vi "Create DSF UDP Loopback Configuration Files.vi"() -> ()   [LabVIEW 2021]
uses:
  Includes/DSF Core.lvlibp/Typedefs/DSF Timing Info.ctl
  Includes/DSF Core.lvlibp/Typedefs/DSF Settings Info.ctl
  Includes/DSF Core.lvlibp/Typedefs/DSF Engine Plugin Thread Configuration.ctl
  Includes/DSF Core.lvlibp/Typedefs/DSF Direction.ctl
  Includes/DSF Core.lvlibp/Typedefs/DSF Byte Order.ctl
  Includes/DSF Core.lvlibp/Typedefs/DSF Data Type.ctl
  Includes/DSF Core.lvlibp/Typedefs/DSF Engine Channel Configuration.ctl
  Includes/DSF Core.lvlibp/Typedefs/DSF Engine Transfer Configuration.ctl
  Includes/DSF Core.lvlibp/Typedefs/DSF Timeout Behavior.ctl
  Includes/DSF Core.lvlibp/Typedefs/DSF Engine Transfer Group Configuration.ctl
  Includes/DSF Core.lvlibp/Typedefs/DSF Engine Plugin Configuration.ctl
  Includes/DSF Core.lvlibp/Typedefs/DSF Engine Framework Configuration.ctl
  Includes/DSF Core.lvlibp/Typedefs/Core Channel Configuration.ctl
  Includes/DSF Core.lvlibp/Typedefs/Core Transfer Configuration.ctl
  Includes/DSF Core.lvlibp/Typedefs/Core Group Configuration.ctl
  Includes/DSF Core.lvlibp/Typedefs/Core Thread Configuration.ctl
  Includes/DSF Core.lvlibp/Typedefs/Core Plugin Configuration.ctl
panel:
  in  "Tx Ports":u16[](array[numeric])
  in  "Rx Ports":u16[](array[numeric])
  out "Framework Configuration":T1
  in  "channels data type":T16=enum."SGL"
  in  "channel count per transfer":u64=1000
  in  "Destination IP Address":string="localhost"
  in  "Source IP Address":string="localhost"
  in  "Local Ports":u16[](array[numeric])
  out "error out":errorcluster
  in  "error in (no error)":errorcluster
  in  "Output Folder":path
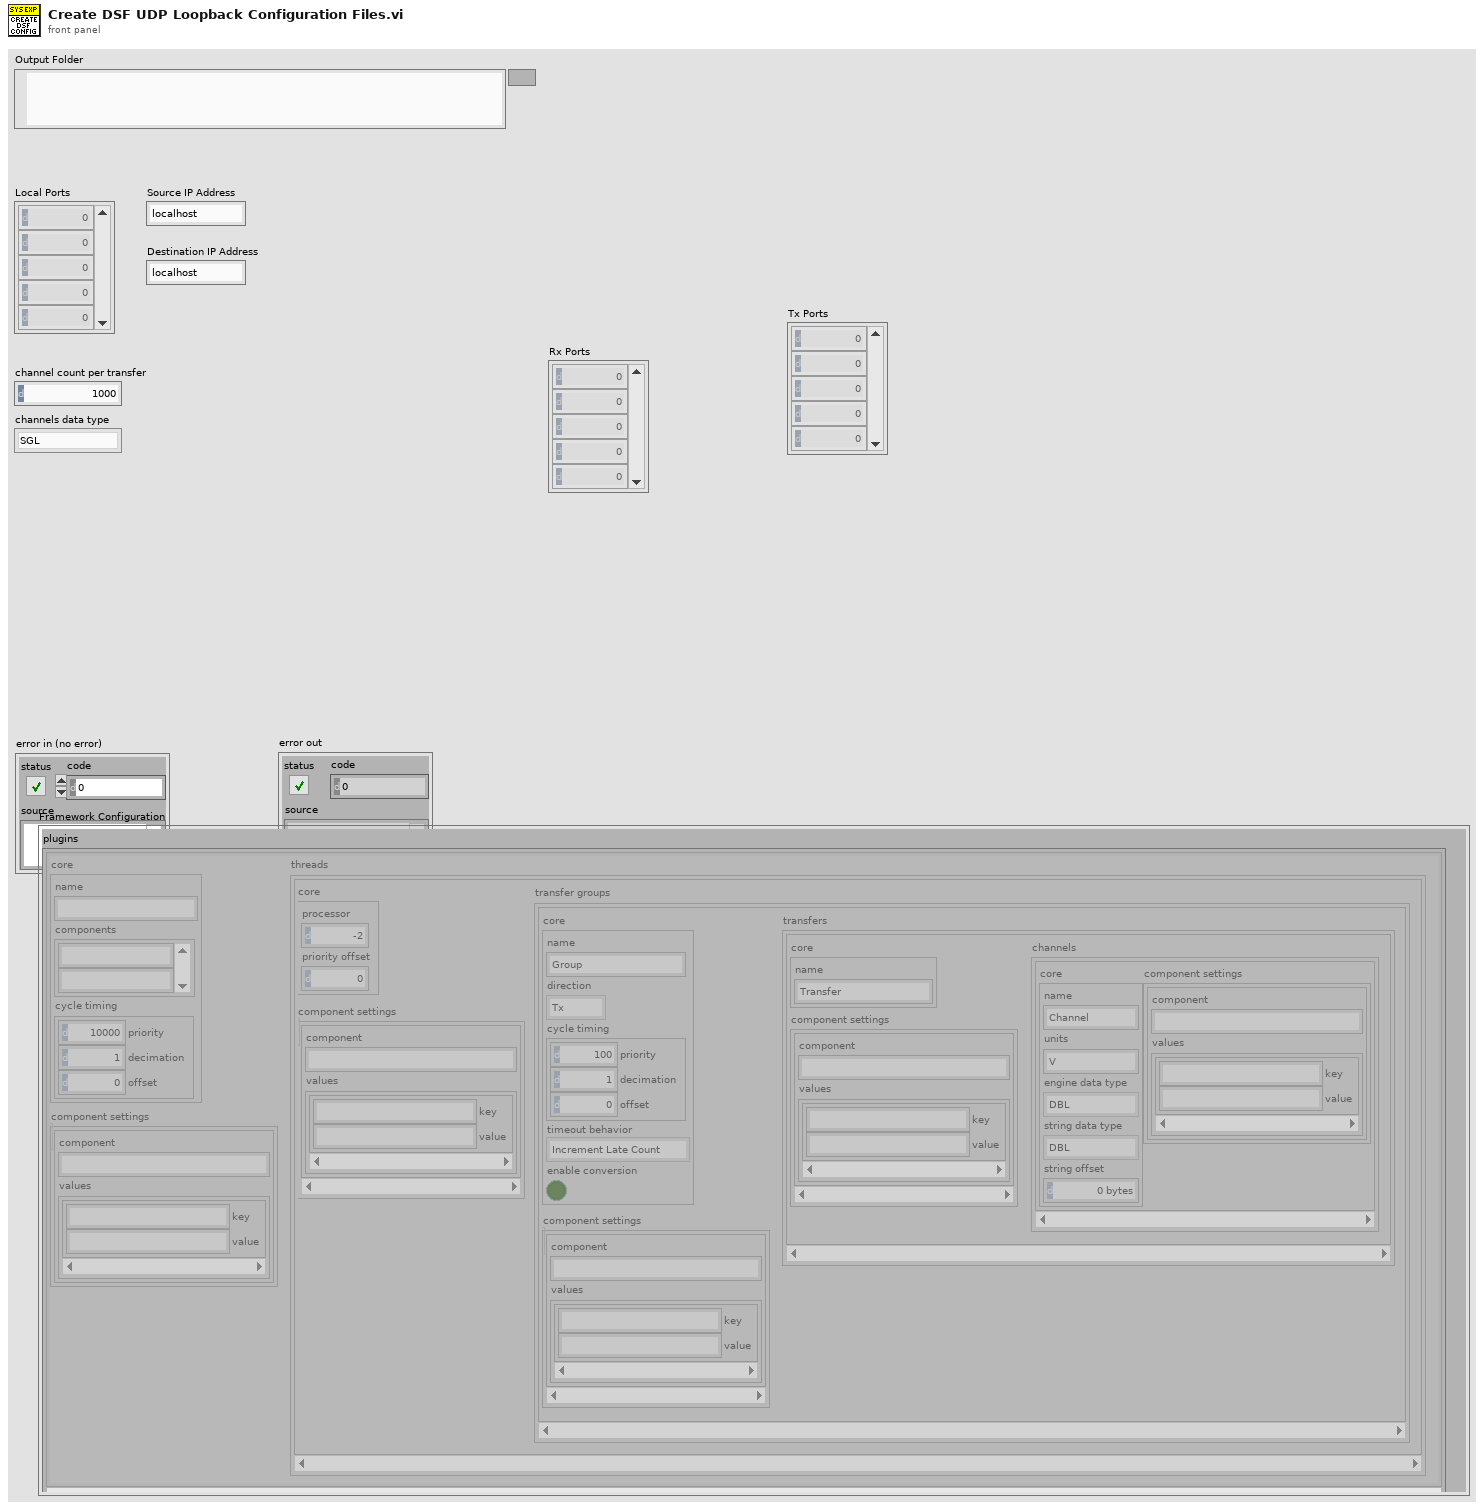
[diagram p1: front panel]
types:
  T1 = typedef "DSF Core.lvlibp/DSF Engine Framework Configuration.ctl" = cluster{"plugins":T2[]}
  T2 = typedef "DSF Core.lvlibp/DSF Engine Plugin Configuration.ctl" = cluster{"core":T3, "component settings":T5[], "threads":T6[]}
  T3 = typedef "DSF Core.lvlibp/Plugin Configuration.lvclass/Core Plugin Configuration.ctl" = cluster{"name":string, "components":string[], "cycle timing":T4}
  T4 = typedef "DSF Core.lvlibp/DSF Timing Info.ctl" = cluster{"priority":u64, "decimation":u64, "offset":u64}
  T5 = typedef "DSF Core.lvlibp/DSF Settings Info.ctl" = cluster{"component":string, "values":cluster{"key":string, "value":string}[]}
  T6 = typedef "DSF Core.lvlibp/DSF Engine Plugin Thread Configuration.ctl" = cluster{"core":T7, "component settings":T5[], "transfer groups":T8[]}
  T7 = typedef "DSF Core.lvlibp/Thread Configuration.lvclass/Core Thread Configuration.ctl" = cluster{"processor":i32, "priority offset":i16}
  T8 = typedef "DSF Core.lvlibp/DSF Engine Transfer Group Configuration.ctl" = cluster{"core":T9, "component settings":T5[], "transfers":T12[]}
  T9 = typedef "DSF Core.lvlibp/Group Configuration.lvclass/Core Group Configuration.ctl" = cluster{"name":string, "direction":T10, "cycle timing":T4, "timeout behavior":T11, "enable conversion":bool}
  T10 = typedef "DSF Core.lvlibp/DSF Direction.ctl" = enum8{"Tx", "Rx"}
  T11 = typedef "DSF Core.lvlibp/DSF Timeout Behavior.ctl" = enum8{"Increment Late Count", "Throw Error"}
  T12 = typedef "DSF Core.lvlibp/DSF Engine Transfer Configuration.ctl" = cluster{"core":T13, "component settings":T5[], "channels":T14[]}
  T13 = typedef "DSF Core.lvlibp/Transfer Configuration.lvclass/Core Transfer Configuration.ctl" = cluster{"name":string}
  T14 = typedef "DSF Core.lvlibp/DSF Engine Channel Configuration.ctl" = cluster{"core":T15, "component settings":T5[]}
  T15 = typedef "DSF Core.lvlibp/Channel Configuration.lvclass/Core Channel Configuration.ctl" = cluster{"name":string, "units":string, "engine data type":T16, "string data type":T16, "string offset":u64}
  T16 = typedef "DSF Core.lvlibp/DSF Data Type.ctl" = enum8{"Bool", "SGL", "DBL", "I8", "I16", "I32", "I64", "U8", "U16", "U32", "U64"}
  T17 = typedef "DSF Core.lvlibp/DSF Engine Plugin Configuration.ctl" = cluster{"name":string, "components":string[], "cycle timing":T4, "threads":T6[], "Transfer Groups":T8[], "settings":T5}
  T18 = typedef "DSF Core.lvlibp/DSF Engine Framework Configuration.ctl" = cluster{"components directory":path, "Plugins":T17[]}
  T19 = typedef "DSF Core.lvlibp/DSF Engine Channel Configuration.ctl" = cluster{"string offset":u64, "string data type":T16, "engine data type":T16, "name":string, "settings":T5}
  T20 = typedef "DSF Core.lvlibp/DSF Byte Order.ctl" = enum8{"big-endian", "little-endian"}
  T21 = typedef "DSF Core.lvlibp/DSF Engine Transfer Group Configuration.ctl" = cluster{"name":string, "direction":T10, "cycle timing":T4, "thread index":i32, "settings":T5, "Transfers":T12[], "timeout behavior":T11}
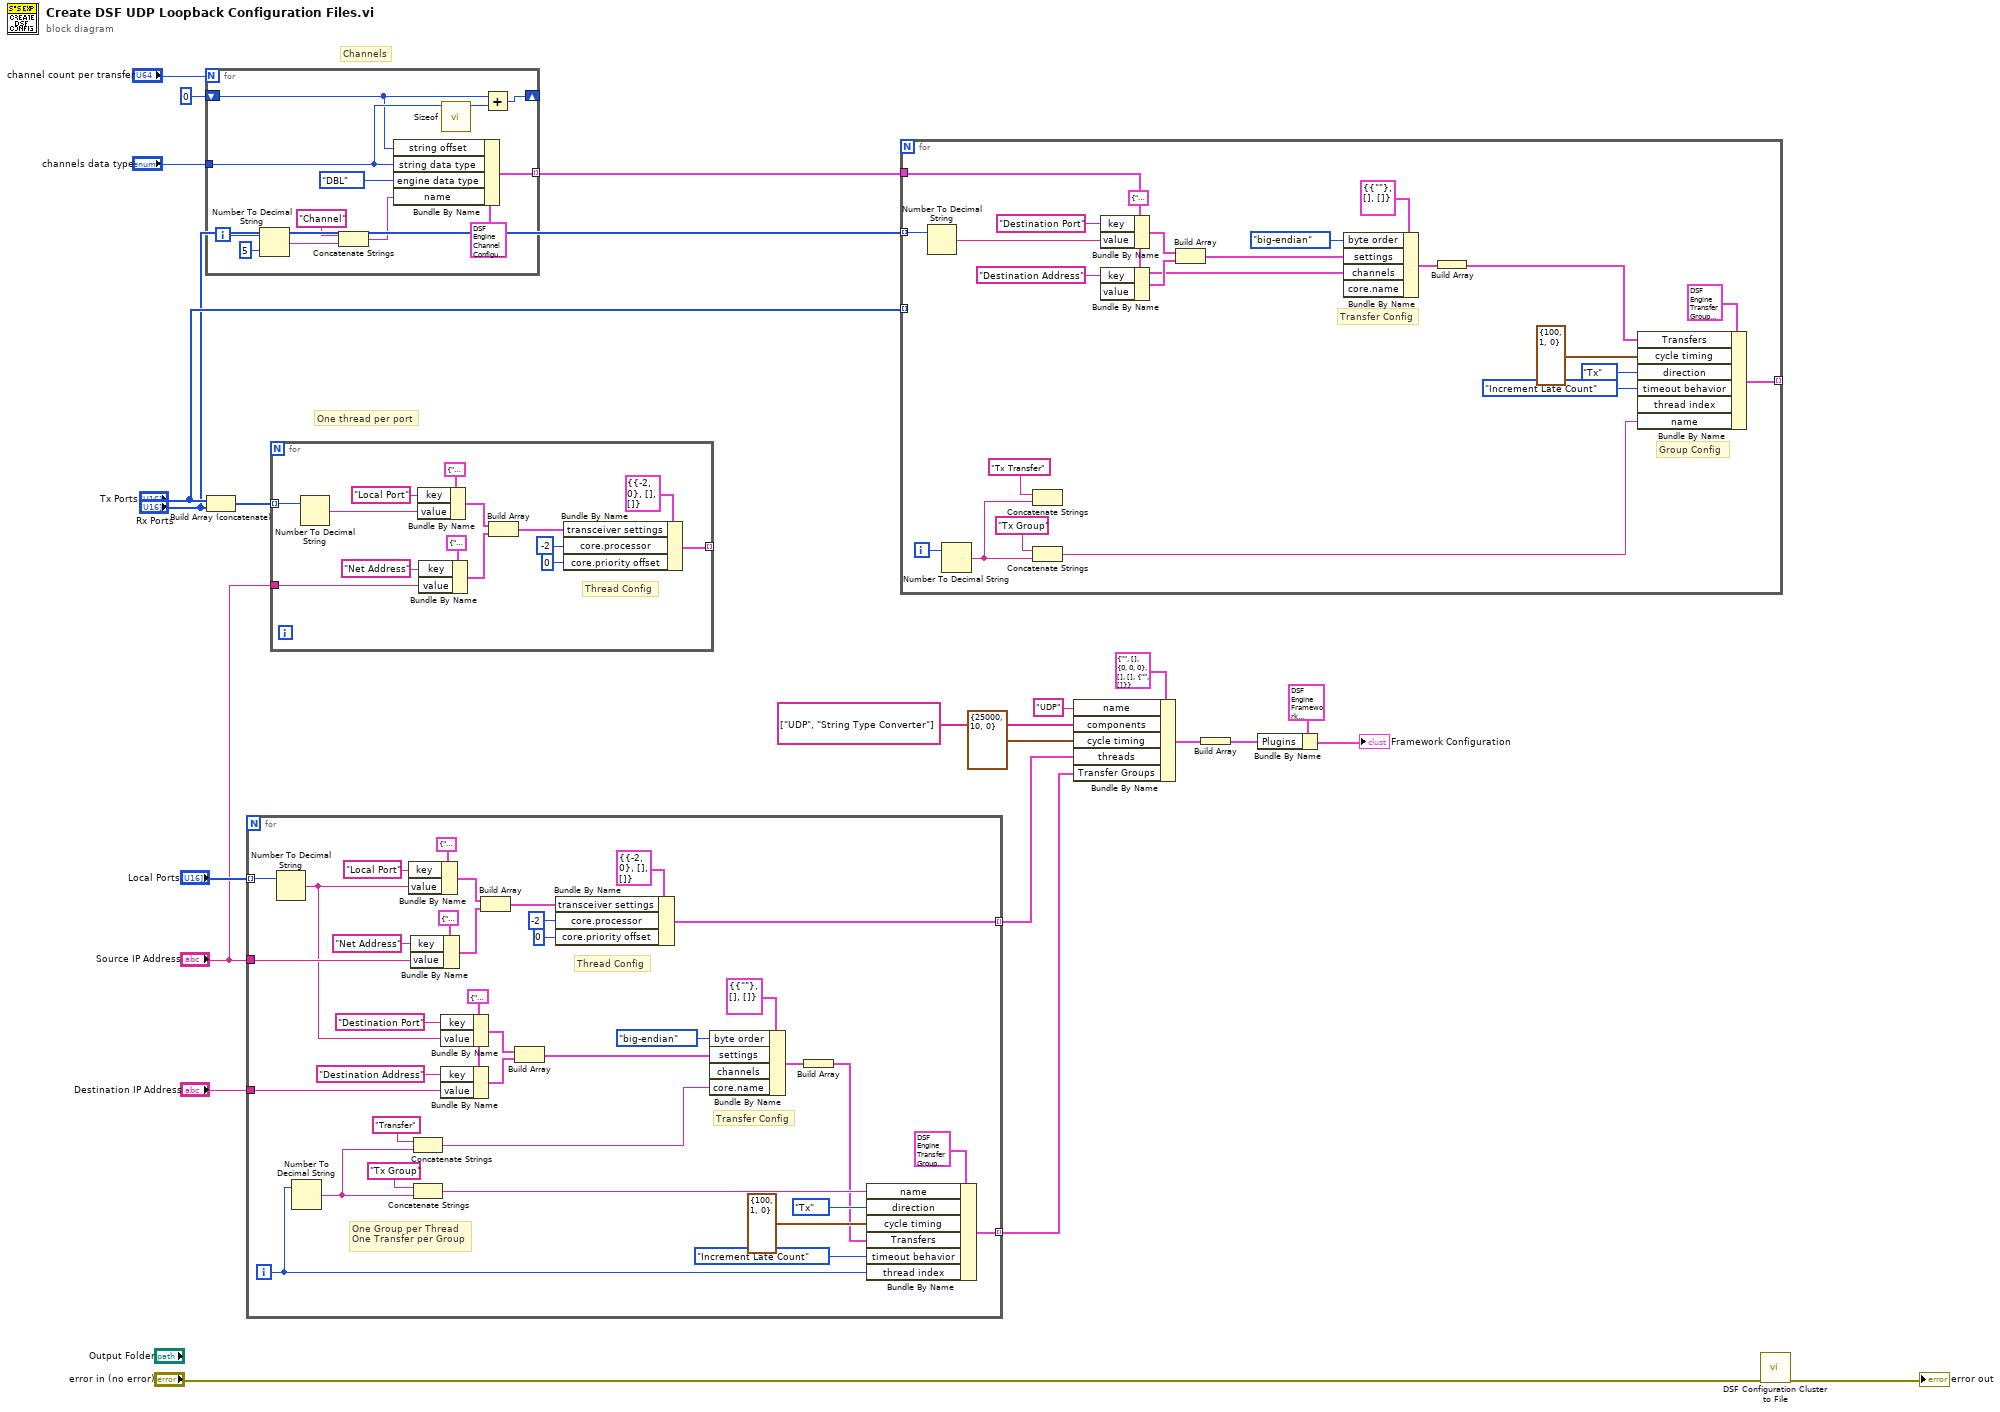
[diagram p0: block diagram]
diagram:
  # "Channels"
  # "One thread per port"
  n1 = for {
    N: "channel count per transfer" -> [_]
    tunnel: "channels data type" -> [w32]
    shift-right: [w24] -> _
    shift-left: u64 0 ("string offset") -> [w25]
    tunnel: [w23] -> w2 mode=indexing
    i -> [w30]
    n2 = Number To Decimal String(number=w30, width (-)=i16 5) -> (decimal integer string=w28:string)
    n3 = Concatenate Strings("Channel" ("name"), w28) -> (w27:string)
    n4 = Bundle By Name(cluster=T19 {"string offset"=0, "string data type"=enum."Bool", "engine data type"=enum."Bool", "name"="", "settings"={"component"="", "values"=[]}} ("channel configuration"), "string offset"=w25, "string data type"=w32, "engine data type"=DSF_Data_Type."DBL", "name"=w27) -> (w23:T19)
    n5 = call "Sizeof.vi"("data type"=w32) -> ("size in bytes"=w26:u64)  [unwired: 9 in, 1 out]
    n6 = Add(x=w25, y=w26) -> (x+y=w24:u64)
  }
  n7 = Build Array (concatenate)("Tx Ports", "Rx Ports") -> (w8:u16[])
  n8 = for {
    tunnel: "Local Ports" -> [w60] mode=indexing
    tunnel: [w59] -> w14 mode=indexing
    tunnel: "Source IP Address" -> [w58]
    tunnel: [w49] -> w13 mode=indexing
    tunnel: "Destination IP Address" -> [w40]
    i -> [w52]
    w46 = cluster{"key":string, "value":string} {"key"="Local Port", "value"="50000"} ("setting")
    # "Group Config"
    # "Transfer Config"
    # "One Group per Thread\nOne Transfer per Group"
    # "Thread Config"
    n9 = Number To Decimal String(number=w60) -> (decimal integer string=w41:string)  [unwired: 1 in]
    n10 = Number To Decimal String(number=w52) -> (decimal integer string=w35:string)  [unwired: 1 in]
    n11 = Bundle By Name(cluster=cluster{"key":string, "value":string} {"key"="Local Port", "value"="50000"} ("setting"), "key"="Local Port", "value"=w41) -> (w63:cluster{"key":string, "value":string})
    n12 = Bundle By Name(cluster=cluster{"key":string, "value":string} {"key"="Local Port", "value"="50000"} ("setting"), "key"="Net Address", "value"=w58) -> (w62:cluster{"key":string, "value":string})
    n13 = Concatenate Strings("Transfer" ("name"), w35) -> (w36:string)
    n14 = Concatenate Strings("Tx Group" ("name"), w35) -> (w45:string)
    n15 = Bundle By Name(cluster=w46, "key"="Destination Port", "value"=w41) -> (w42:cluster{"key":string, "value":string})
    n16 = Bundle By Name(cluster=w46, "key"="Destination Address", "value"=w40) -> (w43:cluster{"key":string, "value":string})
    n17 = Build Array(w63, w62) -> (w61:cluster{"key":string, "value":string}[])
    n18 = Build Array(w42, w43) -> (w39:cluster{"key":string, "value":string}[])
    n19 = Bundle By Name(cluster=T6 {"core"={"processor"=-2, "priority offset"=0}, "component settings"=[], "transfer groups"=[]} ("threads"), "transceiver settings"=w61, "core.processor"=-2 ("processor"), "core.priority offset"=i16 0 ("priority offset")) -> (w59:T6)
    n20 = Bundle By Name(cluster=T12 {"core"={"name"=""}, "component settings"=[], "channels"=[]} ("Transfer Configuration"), "byte order"=DSF_Byte_Order."big-endian", "settings"=w39, "core.name"=w36) -> (w38:T12)  [unwired: 1 in]
    n21 = Build Array(w38) -> (w37:T12[])
    n22 = Bundle By Name(cluster=T21 {"name"="", "direction"=enum."Tx", "cycle timing"={"priority"=0, "decimation"=0, "offset"=0}, "thread index"=0, "settings"={"component"="", "values"=[]}, "Transfers"=[], "timeout behavior"=enum."Increment Late Count"} ("Transfer Group Configuration"), "name"=w45, "direction"=DSF_Direction."Tx", "cycle timing"=T4 {"priority"=100, "decimation"=1, "offset"=0}, "Transfers"=w37, "timeout behavior"=DSF_Timeout_Behavior."Increment Late Count", "thread index"=w52) -> (w49:T21)
  }
  n23 = for {
    tunnel: w8 -> [w74] mode=indexing
    tunnel: [w73] -> _ mode=indexing
    tunnel: "Source IP Address" -> [w72]
    # "Thread Config"
    n24 = Number To Decimal String(number=w74) -> (decimal integer string=w71:string)  [unwired: 1 in]
    n25 = Bundle By Name(cluster=cluster{"key":string, "value":string} {"key"="Local Port", "value"="50000"} ("setting"), "key"="Local Port", "value"=w71) -> (w77:cluster{"key":string, "value":string})
    n26 = Bundle By Name(cluster=cluster{"key":string, "value":string} {"key"="Local Port", "value"="50000"} ("setting"), "key"="Net Address", "value"=w72) -> (w76:cluster{"key":string, "value":string})
    n27 = Build Array(w77, w76) -> (w75:cluster{"key":string, "value":string}[])
    n28 = Bundle By Name(cluster=T6 {"core"={"processor"=-2, "priority offset"=0}, "component settings"=[], "transfer groups"=[]} ("threads"), "transceiver settings"=w75, "core.processor"=-2 ("processor"), "core.priority offset"=i16 0 ("priority offset")) -> (w73:T6)
  }
  n29 = for {
    tunnel: "Tx Ports" -> [_] mode=indexing
    tunnel: [w100] -> _ mode=indexing
    tunnel: w2 -> [w90]
    tunnel: "Rx Ports" -> [w86] mode=indexing
    i -> [w104]
    w93 = cluster{"key":string, "value":string} {"key"="Local Port", "value"="50000"} ("setting")
    # "Transfer Config"
    # "Group Config"
    n30 = Number To Decimal String(number=w86) -> (decimal integer string=w85:string)  [unwired: 1 in]
    n31 = Number To Decimal String(number=w104) -> (decimal integer string=w88:string)  [unwired: 1 in]
    n32 = Concatenate Strings("Tx Transfer" ("name"), w88) -> ()  [unwired: 1 out]
    n33 = Concatenate Strings("Tx Group" ("name"), w88) -> (w103:string)
    n34 = Bundle By Name(cluster=w93, "key"="Destination Port", "value"=w85) -> (w97:cluster{"key":string, "value":string})
    n35 = Bundle By Name(cluster=w93, "key"="Destination Address") -> (w96:cluster{"key":string, "value":string})  [unwired: 1 in]
    n36 = Build Array(w97, w96) -> (w98:cluster{"key":string, "value":string}[])
    n37 = Bundle By Name(cluster=T12 {"core"={"name"=""}, "component settings"=[], "channels"=[]} ("Transfer Configuration"), "byte order"=DSF_Byte_Order."big-endian", "settings"=w98, "channels"=w90) -> (w99:T12)  [unwired: 1 in]
    n38 = Build Array(w99) -> (w87:T12[])
    n39 = Bundle By Name(cluster=T21 {"name"="", "direction"=enum."Tx", "cycle timing"={"priority"=0, "decimation"=0, "offset"=0}, "thread index"=0, "settings"={"component"="", "values"=[]}, "Transfers"=[], "timeout behavior"=enum."Increment Late Count"} ("Transfer Group Configuration"), "Transfers"=w87, "cycle timing"=T4 {"priority"=100, "decimation"=1, "offset"=0}, "direction"=DSF_Direction."Tx", "timeout behavior"=DSF_Timeout_Behavior."Increment Late Count", "name"=w103) -> (w100:T21)  [unwired: 1 in]
  }
  n40 = Bundle By Name(cluster=T17 {"name"="", "components"=[], "cycle timing"={"priority"=0, "decimation"=0, "offset"=0}, "threads"=[], "Transfer Groups"=[], "settings"={"component"="", "values"=[]}} ("Plugin Configuration"), "name"="UDP", "components"=string[] ["UDP", "String Type Converter"], "cycle timing"=T4 {"priority"=25000, "decimation"=10, "offset"=0}, "threads"=w14, "Transfer Groups"=w13) -> (w12:T17)
  n41 = Build Array(w12) -> (w11:T17[])
  n42 = Bundle By Name(cluster=T18 {"components directory"=path "", "Plugins"=[{"name"="UDP", "components"=["UDP", "String Type Converter"], "cycle timing"={"priority"=25000, "decimation"=10, "offset"=0}, "threads"=[], "Transfer Groups"=[], "settings"={"component"="", "values"=[]}}]} ("framework configuration"), "Plugins"=w11) -> (→"Framework Configuration":T18)
  n43 = call "DSF Configuration Cluster to File.vi"("error in (no error)"="error in (no error)") -> ("error out"=→"error out":errorcluster)  [unwired: 9 in, 1 out]
